vi "Run.vi"(4 "Dispense?":bool, 6 "Pickup_Test_Number":dbl, 8 "error in (no error)":errorcluster, 9 "Assembly Type":string, 10 "Control In":T1={"I-O.lvclass"=refnum, "Gantry"=refnum, "Dispenser"="COM1"}, 11 "Assembly In":refnum<class "Assembly Run.lvclass">) -> (0 "error out":errorcluster, 2 "Control Out":T1={"I-O.lvclass"=refnum, "Gantry"=refnum, "Dispenser"="COM1"}, 3 "Assembly Out":refnum<class "Assembly Run.lvclass">)   [LabVIEW 2021, in "Assembly Run.lvclass"]
uses:
  Assembly Run.lvclass
  Controller/Controllers.ctl
  Controller/I-O/I-O.lvclass
  C:/Program Files (x86)/Aerotech/A3200/LabVIEW/2010/Bin/Aerotech.A3200.dll
  Program Files (x86)/Aerotech/A3200/LabVIEW/2010/Bin/Aerotech.A3200.dll
  Assembly Run.lvclass/Assembly Run.ctl
  Workspace/Fixture.lvclass/Fixture.ctl
  Workspace/Fixture.lvclass
  Routine/Routine.lvclass
  Controller/Motion/Motion.lvclass
  Controller/Controller.lvclass
panel:
  out "Numeric 4":i32
  out "Numeric 3":i32
  out "Numeric 2":i32
  out "Numeric":i32
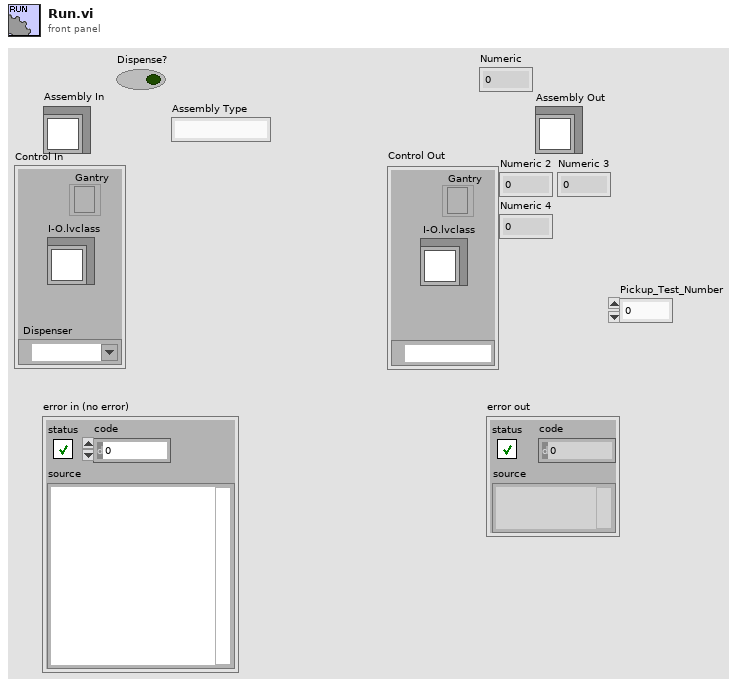
[diagram p1: front panel]
types:
  T1 = typedef "Controller.lvclass/Controllers.ctl" = cluster{"I-O.lvclass":refnum<class "I-O.lvclass">, "Gantry":refnum<k24>, "Dispenser":refnum<visa-resource-name>}
  T2 = typedef "Fixture.lvclass/Workspace.ctl" = cluster{"XYZTheta":dbl[], "Workspace Valve":i32, "Workspace Sensor":i32}
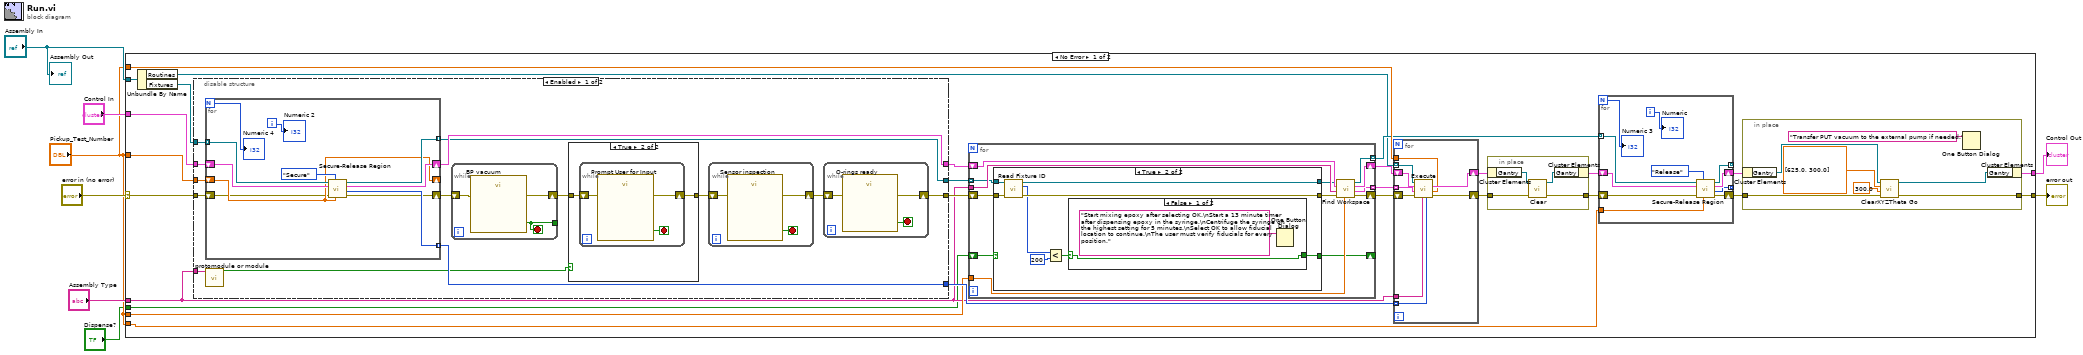
[diagram p0: block diagram]
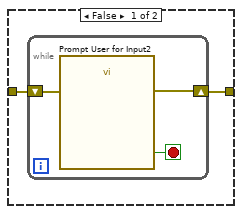
[diagram p4: hidden frame]
diagram:
  n1 = case shown="No Error" "error in (no error)" {
    selector: "error in (no error)" -> [w18 w141]
    tunnel: [w12 w141] -> w7
    tunnel: [w19 w140] -> w6
    tunnel: "Assembly In" -> [w31 _]
    tunnel: "Control In" -> [w28 w140]
    tunnel: "Assembly Type" -> [w10 _]
    tunnel: "Pickup_Test_Number" -> [w25 _]
    tunnel: "Pickup_Test_Number" -> [w23 _]
    tunnel: "Pickup_Test_Number" -> [w24 _]
    tunnel: "Pickup_Test_Number" -> [w22 _]
    tunnel: "Dispense?" -> [w9 _]
    frame No Error {
      n2 = Unbundle By Name(w31) -> ("Routines"=w11:refnum<class "Routine.lvclass">[], "Fixtures"=w32:refnum<class "Fixture.lvclass">[])
      n3 = disable-structure shown="Enabled" {
        disable-tunnel: [w73 w115] -> w34
        disable-tunnel: w32 -> [w83 w115]
        disable-tunnel: w28 -> [w82 w114]
        disable-tunnel: [w81 w114] -> w27
        disable-tunnel: [w80 _] -> w26
        disable-tunnel: w23 -> [w79 _]
        disable-tunnel: w18 -> [w78 _]
        disable-tunnel: [w70 _] -> w17
        disable-tunnel: w10 -> [w72 _]
        frame Enabled {
          n4 = for {
            N -> [w105]
            tunnel: [w113] -> w73 mode=indexing
            tunnel: w83 -> [w112] mode=indexing
            shift-right: [w110] -> w81
            shift-left: w82 -> [w111]
            tunnel: [w108] -> w80 mode=indexing
            shift-right: [w107] -> _
            shift-left: w79 -> [w107]
            shift-right: [w104] -> w77
            shift-left: w78 -> [w103]
            i -> [w106]
            n5 = call-dynamic "Secure-Release Region.vi"("Test Run Number"=w107, "Action"=enum16{"Secure", "Release"}."Secure", "error in (no error)"=w103, "Control In"=w111, "Fixture in"=w112) -> ("error out"=w104:errorcluster, "Position"=w108:i32, "Control Out"=w110:T1, "Fixture out"=w113:refnum<class "Fixture.lvclass">)  [unwired: 3 in]
            "Numeric 2" <- w106
            "Numeric 4" <- w105
          }
          n6 = call "protomodule or module.vi"("assembly type"=w72) -> ("protomodule? (T)"=w76:bool)  [unwired: 10 in]
          n7 = while {
            tunnel: [w102] -> _
            shift-right: [w100] -> w75
            shift-left: w77 -> [w101]
            stop <- w102 stop-if-true
            n8 = call "BP vacuum"("error in (no error)"=w101) -> ("BP vacuum is on?"=w102:bool, "error out"=w100:errorcluster)  [unwired: 16 in, 1 out]
          }
          n9 = case shown="True" w76 {
            tunnel: w75 -> [w91 w96]
            tunnel: [w90 w95] -> w74
            frame False {
              n10 = while {
                shift-right: [w93] -> w90
                shift-left: w91 -> [w94]
                stop <- w92 stop-if-true
                n11 = call "Prompt User for Input2"("error in (no error)"=w94) -> ("HB backlighting on?"=w92:bool, "error out"=w93:errorcluster)  [unwired: 16 in, 1 out]
              }
            }
            frame True {
              n12 = while {
                shift-right: [w97] -> w95
                shift-left: w96 -> [w98]
                stop <- w99 stop-if-true
                n13 = call "Prompt User for Input"("error in (no error)"=w98) -> ("BP paper is removed?"=w99:bool, "error out"=w97:errorcluster)  [unwired: 16 in, 1 out]
              }
            }
          }
          n14 = while {
            shift-right: [w85] -> w71
            shift-left: w74 -> [w84]
            stop <- w86 stop-if-true
            n15 = call "Sensor inspection"("error in (no error)"=w84) -> ("Sensors inspected?"=w86:bool, "error out"=w85:errorcluster)  [unwired: 16 in, 1 out]
          }
          n16 = while {
            shift-right: [w88] -> w70
            shift-left: w71 -> [w87]
            stop <- w89 stop-if-true
            n17 = call "O-rings ready"("error in (no error)"=w87) -> ("O-rings ready?"=w89:bool, "error out"=w88:errorcluster)  [unwired: 16 in, 1 out]
          }
        }
        frame Disabled {
        }
      }
      n18 = for {
        tunnel: w34 -> [w41] mode=indexing
        tunnel: [w44] -> w35 mode=indexing
        tunnel: [w48] -> w21 mode=indexing
        shift-right: [w46] -> w30
        shift-left: w27 -> [w47]
        tunnel: w10 -> [w45]
        tunnel: w22 -> [w43]
        shift-right: [w42] -> w16
        shift-left: w17 -> [w39]
        shift-right: [w36] -> _
        shift-left: w9 -> [w37]
        n19 = case shown="True" w37 {
          selector: w37 -> [w49 _]
          tunnel: w41 -> [w51 w59]
          tunnel: [w51 w58] -> w40
          tunnel: w39 -> [w50 w57]
          tunnel: [w50 w56] -> w38
          tunnel: [w49 w52] -> w36
          frame False {
          }
          frame True {
            n20 = call "Read Fixture ID.vi"("error in (no error)"=w57, "Fixture in"=w59) -> ("error out"=w56:errorcluster, "Fixture ID"=w55:i32, "Fixture out"=w58:refnum<class "Fixture.lvclass">)  [unwired: 7 in]
            n21 = Less?(x=w55, y=200) -> (x < y?=w53:bool)
            n22 = case shown="False" w53 {
              selector: w53 -> [w60 w62]
              tunnel: [w60 w62] -> w52
              frame False {
                n23 = One Button Dialog(message="Start mixing epoxy after selecting OK.\nStart a 13 minute timer after dispensing epoxy in the syringe.\nCentrifuge the syringe on the highest setting for 5 minutes.\nSelect OK to allow fiducial location to continue.\nThe user must verify fiducials for every position.") -> ()  [unwired: 1 in, 1 out]
              }
              frame True {
              }
            }
          }
        }
        n24 = call-dynamic "Find Workspace.vi"("Pickup_Test_Number"=w43, "Error In"=w38, "Assembly Type"=w45, "Control In"=w47, "Workspace In"=w40) -> ("Error Out"=w42:errorcluster, 1:"Workspace Out"=w44:T2, "Control Out"=w46:T1, 3:"Workspace Out"=w48:refnum<class "Fixture.lvclass">)  [unwired: 3 in]
      }
      n25 = for {
        tunnel: w11 -> [w139] mode=indexing
        tunnel: w35 -> [w138] mode=indexing
        shift-right: [w136] -> w29
        shift-left: w30 -> [w137]
        tunnel: w10 -> [w135]
        tunnel: w26 -> [w134] mode=indexing
        tunnel: w24 -> [w133]
        shift-right: [w131] -> w15
        shift-left: w16 -> [w132]
        n26 = call-dynamic "Execute.vi"("NumberInput"=w133, "Position"=w134, "Assembly Type"=w135, "error in (no error)"=w132, "Workspace"=w138, "Control In"=w137, "Routine in"=w139) -> ("error out"=w131:errorcluster, "Control Out"=w136:T1)  [unwired: 2 in, 1 out]
      }
      n27 = in-place {
        in-place-border: w15 -> [w128]
        in-place-border: [w127] -> w14
        n28 = in-place-cluster #1(w29) -> ("Gantry"=w129:refnum<k24>)
        n29 = call "Clear.vi"("error in (no error)"=w128, "Gantry In"=w129) -> ("error out"=w127:errorcluster, "Gantry Out"=w130:refnum<k24>)  [unwired: 8 in]
        n30 = in-place-cluster #1("Gantry"=w130) -> (w33:T1)
      }
      n31 = for {
        N -> [w118]
        tunnel: w21 -> [w126] mode=indexing
        shift-right: [w125] -> w20
        shift-left: w33 -> [w124]
        tunnel: w25 -> [w122]
        tunnel: [w120] -> _ mode=indexing
        tunnel: [w119] -> _ mode=indexing
        shift-right: [w116] -> w13
        shift-left: w14 -> [w117]
        i -> [w121]
        n32 = call-dynamic "Secure-Release Region.vi"("Test Run Number"=w122, "Action"=enum16{"Secure", "Release"}."Release", "error in (no error)"=w117, "Control In"=w124, "Fixture in"=w126) -> ("error out"=w116:errorcluster, "Position"=w120:i32, "Control Out"=w125:T1, "Fixture out"=w119:refnum<class "Fixture.lvclass">)  [unwired: 3 in]
        "Numeric" <- w121
        "Numeric 3" <- w118
      }
      n33 = in-place {
        in-place-border: w13 -> [w64]
        in-place-border: [w63] -> w12
        n34 = in-place-cluster #2(w20) -> ("Gantry"=w68:refnum<k24>)
        n35 = call "ClearXYZTheta Go.vi"("error in (no error)"=w64, "Speed"=300.0, "XYZTheta In"=dbl[] [625.0, 300.0], "Gantry In"=w68) -> ("error out"=w63:errorcluster, "Gantry Out"=w67:refnum<k24>)  [unwired: 5 in, 1 out]
        n36 = One Button Dialog(message="Transfer PUT vacuum to the external pump if needed.") -> ()  [unwired: 1 in, 1 out]
        n37 = in-place-cluster #2("Gantry"=w67) -> (w19:T1)
      }
    }
    frame Error {
    }
  }
  "error out" <- w7
  "Control Out" <- w6
  "Assembly Out" <- "Assembly In"
